vi "Configure Multi Eval Meas List Segment Channel Bandwidth.vi"(6 "Channel Bandwidth (20 MHz)":i32(ring)=3 items=["5 MHz", "10 MHz", "15 MHz", "20 MHz", "25 MHz", "30 MHz", "40 MHz", "50 MHz", "60 MHz", "80 MHz", "90 MHz", "100 MHz"], 7 "CC (1)":T1=1, 8 "error in (no error)":errorcluster, 9 "Segment (1)":i32=1, 10 "Instance (1)":T2=1, 11 "VISA resource name":refnum<visa-resource-name>) -> (0 "error out":errorcluster, 3 "VISA resource name out":refnum<visa-resource-name>)   [LabVIEW 2020, in "Rohde&Schwarz CMWXP NR FR1 Measurement.lvlib"]
doc: "Specifies the channel bandwidth of carrier <cc>, used in segment <no>.\n\nAttribute:\nRSCMWXPNRFR1M_ATTR_MULTI_EVAL_MEAS_LIST_SEGMENT_CHANNEL_BANDWIDTH\n\nRemote-control command:\nCONFigure:NRSub:MEAS<i>:LIST:SEGMent<no>[:CC<cc>]:CBANdwidth"
uses:
  <instrlib>/Rohde&Schwarz CMWXP NR FR1 Measurement/Rohde&Schwarz CMWXP NR FR1 Measurement.lvlib
  <instrlib>/Rohde&Schwarz CMWXP NR FR1 Measurement/Private/_Instance.ctl
  <instrlib>/Rohde&Schwarz CMWXP NR FR1 Measurement/Private/_Carrier Component.ctl
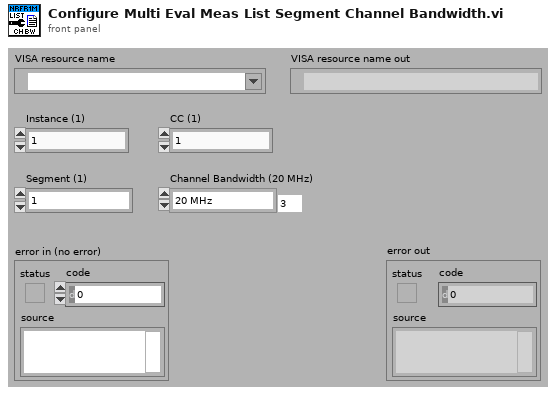
[diagram p1: front panel]
types:
  T1 = typedef "Rohde&Schwarz CMWXP NR FR1 Measurement.lvlib/_Carrier Component.ctl" = i32
  T2 = typedef "Rohde&Schwarz CMWXP NR FR1 Measurement.lvlib/_Instance.ctl" = i32
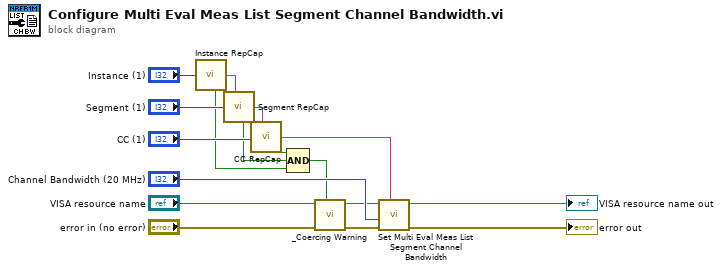
[diagram p0: block diagram]
diagram:
  n1 = call <instrlib>:"Instance RepCap.vi"("Instance In"="Instance (1)") -> ("In Range?"=w8:bool, "RepCap Identifier Out"=w11:string)  [unwired: 1 in]
  n2 = call <instrlib>:"Segment RepCap.vi"("Segment In"="Segment (1)", "RepCap String In (\"\")"=w11) -> ("In Range?"=w7:bool, "RepCap Identifier Out"=w12:string)
  n3 = call <instrlib>:"CC RepCap.vi"("CC In"="CC (1)", "RepCap String In (\"\")"=w12) -> ("In Range?"=w6:bool, "RepCap Identifier Out"=w10:string)
  n4 = Compound Arithmetic op=AND(w6, w7, w8) -> (w1:bool)
  n5 = call <instrlib>:"_Coercing Warning.vi"("In Range?"=w1, "error in (no error)"="error in (no error)", "VISA resource name"="VISA resource name") -> ("error out"=w3:errorcluster, "VISA resource name out"=w2:refnum<visa-resource-name>)  [unwired: 7 in]
  n6 = call "Set Multi Eval Meas List Segment Channel Bandwidth"("Repeated Capabilities"=w10, "error in (no error)"=w3, "Multi Eval Meas List Segment Channel Bandwidth (0 - 5 MHz)"="Channel Bandwidth (20 MHz)", "instrument handle"=w2) -> ("error out"=→"error out":errorcluster, "instrument handle out"=→"VISA resource name out":refnum<visa-resource-name>)  [unwired: 6 in]
